vi "Construct - File (Binary).vi"(10 "section":string, 11 "config file":path) -> (0 "Error Out":errorcluster, 3 "Text File":refnum<class "Text File - Binary.lvclass">)   [LabVIEW 2019, in "TSC Event Logger.lvlib" / "Text File - Binary.lvclass"]
doc: "Constructor for a binary file type - from read of common ini format.\n\n<b>Code Developed By:</b>\nTechnology Service Corporation\nBloomington, IN 47403\nwww.tsc.com/atcs\n\nDeveloper:\nDaniel Coons"
uses:
  Text File - Binary.lvclass
  C:/Development/Open Source/tsc-event-logger/Log Sinks/Text File/Text File.lvclass
  Text File/Text File.lvclass
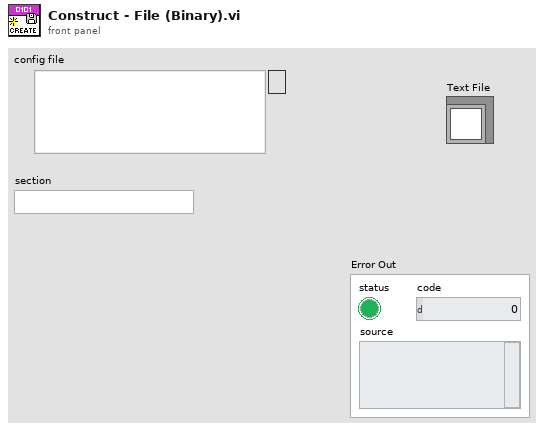
[diagram p1: front panel]
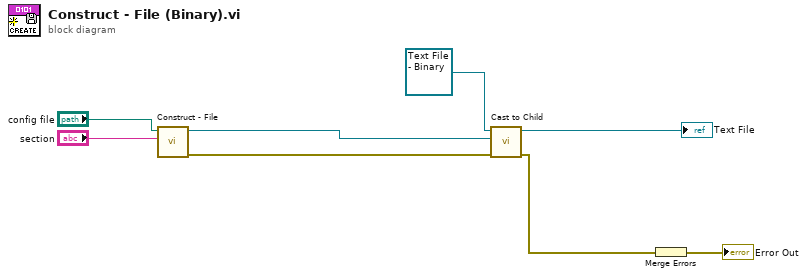
[diagram p0: block diagram]
diagram:
  n1 = call "Construct - File.vi"("section"="section", "config file"="config file") -> ("Error Out"=w2:errorcluster, "Text File"=w3:refnum<class "Text File.lvclass">)  [unwired: 8 in]
  n2 = call "Cast to Child.vi"("error in (no error)"=w2, "Parent"=w3, "Child in"=refnum<class "Text File - Binary.lvclass"> refnum ("TSC Event Logger.lvlib:Text File - Binary.lvclass")) -> ("error out"=w1:errorcluster, "Child Out"=→"Text File":refnum<class "Text File - Binary.lvclass">)  [unwired: 7 in]
  n3 = Merge Errors(w1) -> (→"Error Out":errorcluster)
